vi "Example - Sort 2D String Array.vi"() -> ()   [LabVIEW 2009, in "xijk_select_best_filter.lvlib"]
doc: "This example VI demonstrates how you can use the Sort 2D String Array VI in your application.\n\nThe Sort 2D String Array VI is useful when you need to sort a 2D array of strings that contains plain text strings and strings representing real numbers. \n\nThis example VI enables the user to perform a multi-column sort on an array of strings by specifying the columns to sort by. The result of the specified sort is returned to the front panel.\n\n<B>Developed by:</B>\n\nMark Ridgley\nmark.ridgley@logicpd.com"
uses:
  xijk_select_best_filter.lvlib
  _TypeDefs/TYPE - Input Array Contains Header Row.ctl
  _TypeDefs/TYPE - Sort Ascending.ctl
panel:
  in  "Stop":bool
  in  "Sort":bool
  out "Sorted Array":string[][](table)
  out "Auto-Generated Array To Sort":string[][](table)
  in  "Preview sorted data":bool
  in  "Sort ascending":T1
  in  "Input array contains header row":T2
  in  "Output columns in sort order":bool
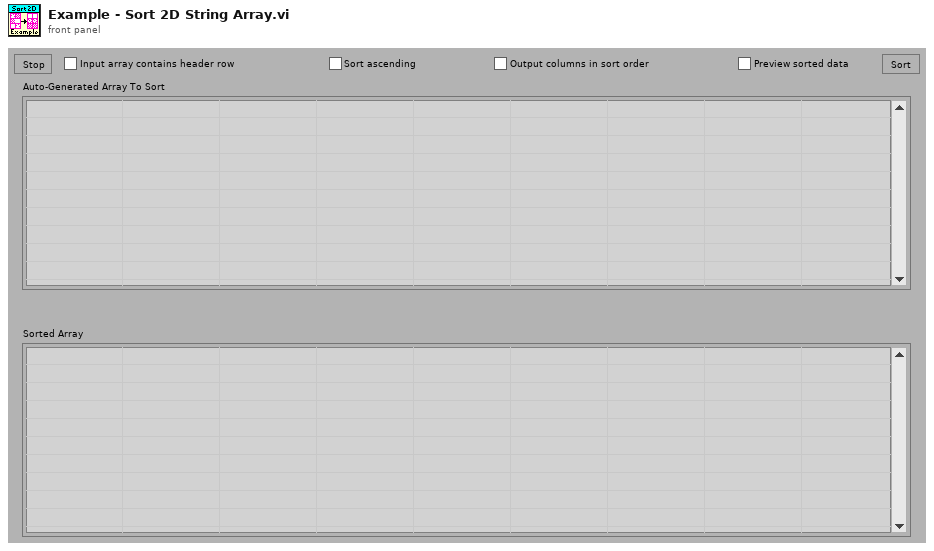
[diagram p1: front panel]
types:
  T1 = typedef "xijk_select_best_filter.lvlib/TYPE - Sort Ascending.ctl" = bool
  T2 = typedef "xijk_select_best_filter.lvlib/TYPE - Input Array Contains Header Row.ctl" = bool
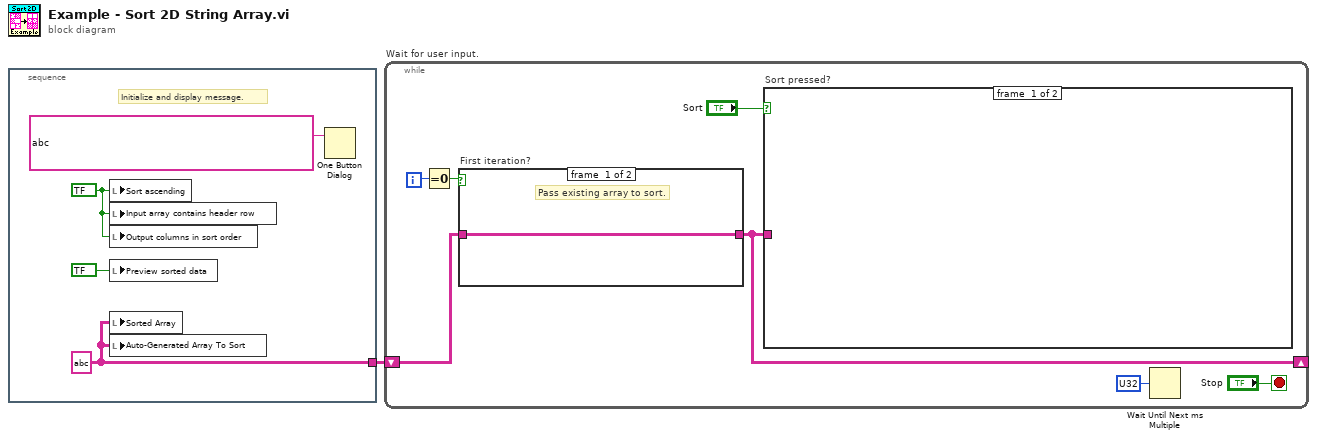
[diagram p0: block diagram]
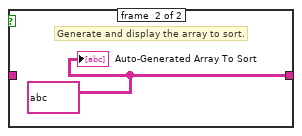
[diagram p2: hidden frame]
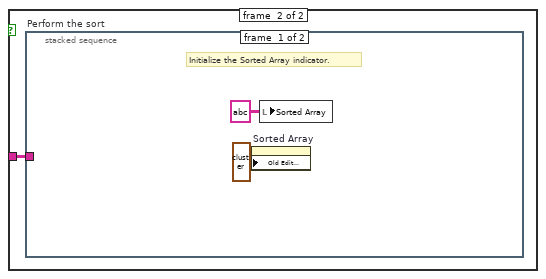
[diagram p3: hidden frame]
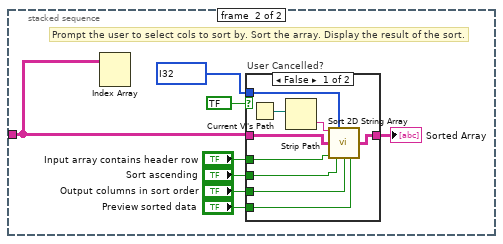
[diagram p4: hidden frame]
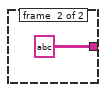
[diagram p5: hidden frame]
diagram:
  n1 = stacked-sequence {
    tunnel: [w3] -> w1
    frame #0 {
      w2 = bool ? ("Sort ascending")
      w3 = string[][] ? ("Array")
      # "Initialize and display message."
      n2 = local write "Sort ascending"(w2) -> ()
      n3 = local write "Input array contains header row"(w2) -> ()
      n4 = local write "Output columns in sort order"(w2) -> ()
      n5 = local write "Preview sorted data"(bool ? ("Preview sorted data")) -> ()
      n6 = local write "Sorted Array"(w3) -> ()
      n7 = local write "Auto-Generated Array To Sort"(w3) -> ()
      n8 = One Button Dialog(message=string ?) -> ()  [unwired: 2 out]
    }
  }
  n9 = while "Wait for user input." {
    shift-right: [w8] -> _
    shift-left: w1 -> [w7]
    i -> [w9]
    stop <- "Stop" stop-if-true
    n10 = Equal To 0?(x=w9) -> (x = 0?=w10:bool)
    n11 = case "First iteration?" shown="True" w10 {
      tunnel: [w13 w14] -> w8
      tunnel: w7 -> [w13 _]
      frame #0 {
        # "Pass existing array to sort."
      }
      frame #1 {
        w14 = string[][] ? ("Auto-Generated Array To Sort")
        # "Generate and display the array to sort."
        "Auto-Generated Array To Sort" <- w14
      }
    }
    n12 = case "Sort pressed?" shown="True" "Sort" {
      tunnel: w8 -> [_ w15]
      frame #0 {
      }
      frame #1 {
        n13 = stacked-sequence "Perform the sort" {
          tunnel: w15 -> [_ w22]
          frame #0 {
            # "Initialize the Sorted Array indicator."
            n14 = property on="Sorted Array" class="Tbl (strict)"("Old Edit Position"=cluster{"Row":i32, "Column":i32} ? ("Edit Position")) -> ()  [unwired: 2 in, 2 out]
            n15 = local write "Sorted Array"(string[][] ? ("Sorted Array")) -> ()
          }
          frame #1 {
            # "Prompt the user to select cols to sort by. Sort the array. Display the result of the sort."
            n16 = Index Array(array=w22) -> ()  [unwired: 2 in, 1 out]
            n17 = case "User Cancelled?" shown="False" bool ? {
              tunnel: "Input array contains header row" -> [w30 _]
              tunnel: "Sort ascending" -> [w29 _]
              tunnel: "Output columns in sort order" -> [w28 _]
              tunnel: w22 -> [w31 _]
              tunnel: i32[] ? ("Indices of Selected Items") -> [w33 _]
              tunnel: "Preview sorted data" -> [w27 _]
              tunnel: [w32 string[][] ? ("Output Array")] -> w20
              frame #0 {
                n18 = Current VI's Path() -> (path=w34:path)
                n19 = Strip Path(path=w34) -> (name=w26:string)  [unwired: 1 out]
                n20 = call "Sort 2D String Array.vi"("Calling VI Name"=w26, "Column Sort Order"=w33, "Input Array"=w31, "Input Array Contains Header Row? (T)"=w30, "Sort Ascending? (T)"=w29, "Output Columns in Sort Order? (F)"=w28, "Preview Sorted Data? (F)"=w27) -> ("Output Array"=w32:string[][])  [unwired: 8 out]
              }
              frame #1 {
              }
            }
            "Sorted Array" <- w20
          }
        }
      }
    }
    n21 = Wait Until Next ms Multiple(millisecond multiple=u32 ?) -> ()  [unwired: 1 out]
  }
